vi "Read_SerialData_TermChar.vi"(7 "timeout (50ms)":u32=50, 8 "error in (no error)":errorcluster, 11 "VISA Refnum in":refnum<visa-resource-name>) -> (0 "error out":errorcluster, 2 "StringData":string, 3 "VISA Refnum out":refnum<visa-resource-name>)   [LabVIEW 2023, in "RS232_Device.lvclass"]
uses:
  RS232_Device.lvclass
  <vilib>/Utility/error.llb/Trim Whitespace One-Sided.vi
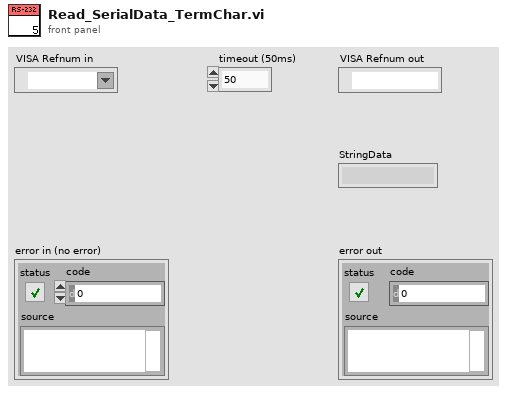
[diagram p1: front panel]
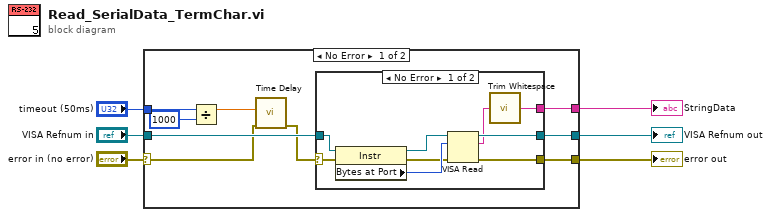
[diagram p0: block diagram]
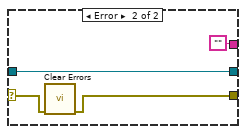
[diagram p2: hidden frame]
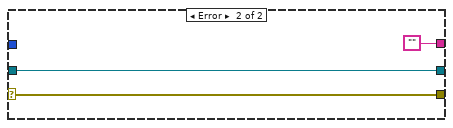
[diagram p3: hidden frame]
diagram:
  n1 = case shown="No Error" "error in (no error)" {
    selector: "error in (no error)" -> [w9 w29]
    tunnel: "VISA Refnum in" -> [w12 w30]
    tunnel: [w15 w30] -> w6
    tunnel: [w14 w29] -> w4
    tunnel: [w13 ""] -> w5
    tunnel: "timeout (50ms)" -> [w11 _]
    frame No Error {
      n2 = Divide(x=w11, y=u32 1000) -> (x/y=w8:dbl)
      n3 = call "Time Delay"("error in (no error)"=w9, "Delay Time (s)"=w8) -> ("error out"=w10:errorcluster)  [unwired: 9 in]
      n4 = case shown="No Error" w10 {
        selector: w10 -> [w20 w28]
        tunnel: w12 -> [w24 w27]
        tunnel: [w18 w27] -> w15
        tunnel: [w19 w25] -> w14
        tunnel: [w16 ""] -> w13
        frame No Error {
          n5 = property class="Instr"(reference=w24, error in=w20) -> (reference out=w23:refnum<visa-resource-name>, error out=w21:errorcluster, "Bytes at Port"=w22:u32)
          n6 = VISA Read(VISA resource name=w23, byte count=w22, error in (no error)=w21) -> (VISA resource name out=w18:refnum<visa-resource-name>, read buffer=w17:string, error out=w19:errorcluster)  [unwired: 1 out]
          n7 = call <vilib>:"Trim Whitespace.vi"("string"=w17) -> ("trimmed string"=w16:string)  [unwired: 1 in]
        }
        frame Error {
          n8 = call <vilib>:"Clear Errors.vi"("error in (no error)"=w28) -> ("error out"=w25:errorcluster)  [unwired: 5 in, 1 out]
        }
      }
    }
    frame Error {
    }
  }
  "VISA Refnum out" <- w6
  "StringData" <- w5
  "error out" <- w4
